vi "SaveTdms.vi"(0 "object in":refnum<class "InstrumentBase.lvclass">, 1 "tdms file":refnum<k34>, 2 "group name":string, 5 "error in (no error)":errorcluster) -> (14 "object out":refnum<class "InstrumentBase.lvclass">, 16 "Channels array":waveform(dbl)[](array[waveform]), 19 "error out":errorcluster)   [LabVIEW 2023, in "InstrumentBase.lvclass"]
uses:
  InstrumentBase.lvclass
  InstrumentBase.lvclass/InstrumentBase.ctl
  <vilib>/measure/NI_MAPro.lvlib
  <vilib>/measure/matone.llb/Extract Single Tone Information 1 Chan.vi
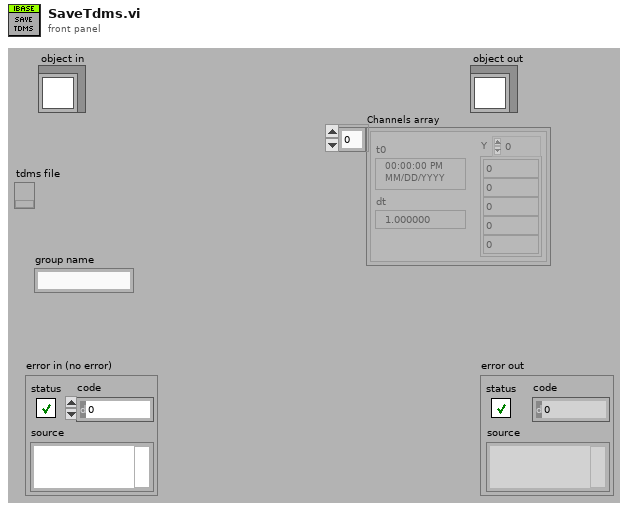
[diagram p1: front panel]
types:
  T1 = cluster{"Config.Ch1.Carrier.Frequency (Hz)":dbl, "Config.Ch2.Carrier.Frequency (Hz)":dbl, "Config.Ch1.Carrier.Amplitude (V)":dbl, "Config.Ch2.Carrier.Amplitude (V)":dbl}
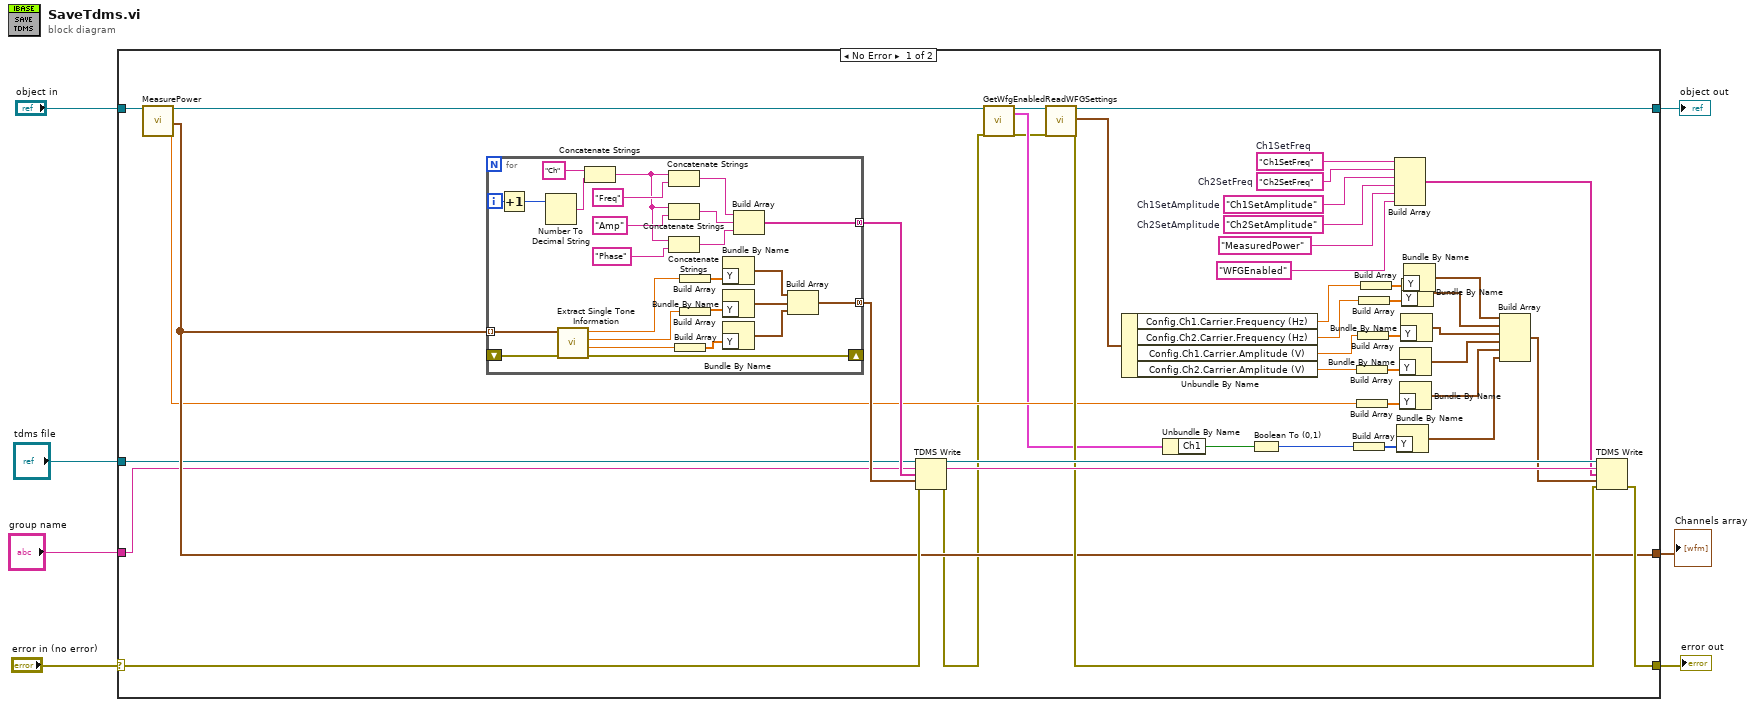
[diagram p0: block diagram]
diagram:
  n1 = case shown="No Error" "error in (no error)" {
    selector: "error in (no error)" -> [w28 w79]
    tunnel: [w24 w79] -> w6
    tunnel: [w27 w78] -> w4
    tunnel: "object in" -> [w23 w78]
    tunnel: "tdms file" -> [w9 _]
    tunnel: "group name" -> [w8 _]
    tunnel: [w21 _] -> w1
    frame No Error {
      w40 = "Ch2SetAmplitude"  # Ch2SetAmplitude
      w42 = "Ch2SetFreq"  # Ch2SetFreq
      w41 = "Ch1SetAmplitude"  # Ch1SetAmplitude
      w43 = "Ch1SetFreq"  # Ch1SetFreq
      n2 = call-dynamic "MeasurePower.vi"("object in"=w23) -> ("object out"=w18:refnum<class "InstrumentBase.lvclass">, "Measured Power"=w20:dbl, "Channels array"=w21:waveform(dbl)[])  [unwired: 13 in, 3 out]
      n3 = for {
        tunnel: [w69] -> w29 mode=concatenating
        shift-right: [w64] -> _
        shift-left: _ -> [w65]
        tunnel: w21 -> [w63] mode=indexing
        tunnel: [w53] -> w30 mode=concatenating
        i -> [w75]
        n4 = Increment(x=w75) -> (x+1=w70:i32)
        n5 = Number To Decimal String(number=w70) -> (decimal integer string=w76:string)  [unwired: 1 in]
        n6 = call-poly <vilib>:"Extract Single Tone Information.vi"("error in (no error)"=w65, "time signal in"=w63) -> ("error out"=w64:errorcluster, "detected phase (deg)"=w58:dbl, "detected amplitude"=w59:dbl, "detected frequency"=w62:dbl)  [unwired: 4 in, 2 out]
        n7 = Concatenate Strings("Ch" ("string"), w76) -> (w68:string)
        n8 = Concatenate Strings(w68, "Freq") -> (w72:string)
        n9 = Concatenate Strings(w68, "Amp") -> (w71:string)
        n10 = Concatenate Strings(w68, "Phase") -> (w66:string)
        n11 = Build Array(w58) -> (w60:dbl[])
        n12 = Build Array(w62) -> (w61:dbl[])
        n13 = Build Array(w59) -> (w57:dbl[])
        n14 = Bundle By Name("Y"=w61) -> (w56:waveform(dbl))  [unwired: 1 in]
        n15 = Bundle By Name("Y"=w57) -> (w55:waveform(dbl))  [unwired: 1 in]
        n16 = Bundle By Name("Y"=w60) -> (w54:waveform(dbl))  [unwired: 1 in]
        n17 = Build Array(w72, w71, w66) -> (w69:string[])
        n18 = Build Array(w56, w55, w54) -> (w53:waveform(dbl)[])
      }
      n19 = TDMS Write(0:w9, 5:w8, 7:w29, 9:w30, 11:w28) -> (4:w32:refnum<k34>, 6:w31:string, 15:w14:errorcluster)  [unwired: 1 in, 1 out]
      n20 = call-dynamic "GetWfgEnabled.vi"("object in"=w18, "error in (no error)"=w14) -> ("object out"=w17:refnum<class "InstrumentBase.lvclass">, "WfgEnabled"=w16:cluster{"Ch1":bool, "Ch2":bool}, "error out"=w15:errorcluster)  [unwired: 15 in]
      n21 = call-dynamic "ReadWFGSettings.vi"("object in"=w17, "error in (no error)"=w15) -> ("object out"=w27:refnum<class "InstrumentBase.lvclass">, "AmplitudeAndVoltage"=w52:T1, "error out"=w22:errorcluster)  [unwired: 15 in]
      n22 = Unbundle By Name(w52) -> ("Config.Ch1.Carrier.Frequency (Hz)"=w47:dbl, "Config.Ch2.Carrier.Frequency (Hz)"=w46:dbl, "Config.Ch1.Carrier.Amplitude (V)"=w45:dbl, "Config.Ch2.Carrier.Amplitude (V)"=w44:dbl)
      n23 = Unbundle By Name(w16) -> ("Ch1"=w12:bool)
      n24 = Boolean To (0,1)(Boolean=w12) -> (0, 1=w11:i16)
      n25 = Build Array(w11) -> (w10:i16[])
      n26 = Build Array(w44) -> (w48:dbl[])
      n27 = Build Array(w20) -> (w35:dbl[])
      n28 = Build Array(w45) -> (w49:dbl[])
      n29 = Build Array(w46) -> (w50:dbl[])
      n30 = Build Array(w47) -> (w51:dbl[])
      n31 = Build Array(w43, w42, w41, w40, "MeasuredPower", "WFGEnabled") -> (w26:string[])
      n32 = Bundle By Name("Y"=w10) -> (w13:waveform(i16))  [unwired: 1 in]
      n33 = Bundle By Name("Y"=w48) -> (w34:waveform(dbl))  [unwired: 1 in]
      n34 = Bundle By Name("Y"=w35) -> (w33:waveform(dbl))  [unwired: 1 in]
      n35 = Bundle By Name("Y"=w49) -> (w37:waveform(dbl))  [unwired: 1 in]
      n36 = Bundle By Name("Y"=w50) -> (w38:waveform(dbl))  [unwired: 1 in]
      n37 = Bundle By Name("Y"=w51) -> (w39:waveform(dbl))  [unwired: 1 in]
      n38 = Build Array(w39, w38, w37, w34, w33, w13) -> (w25:waveform(dbl)[])
      n39 = TDMS Write(0:w32, 5:w31, 7:w26, 9:w25, 11:w22) -> (15:w24:errorcluster)  [unwired: 1 in, 3 out]
    }
    frame Error {
    }
  }
  "error out" <- w6
  "object out" <- w4
  "Channels array" <- w1
